vi "inverse se2.vi"(6 "angle unit":u16(ring) items=["radians", "degree"], 8 "error in (no error)":errorcluster, 11 "T":dbl[][](array[numeric])) -> (0 "Error Out":errorcluster, 1 "theta":dbl, 2 "y":dbl, 3 "x":dbl)   [LabVIEW 2017]
doc: "This function builds and outputs a 3x3 homogeneous transformation as a 2-D array(T). Inputs are horizontal translation (X), vertical translation (Y), and rotation (theta) in radians. The default value of theta is 0 rad."
uses:
  <vilib>/Utility/error.llb/Error Cluster From Error Code.vi
  <vilib>/ErrorRing/Error Ring.xnode
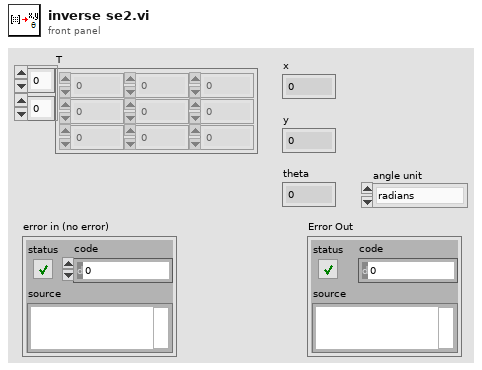
[diagram p1: front panel]
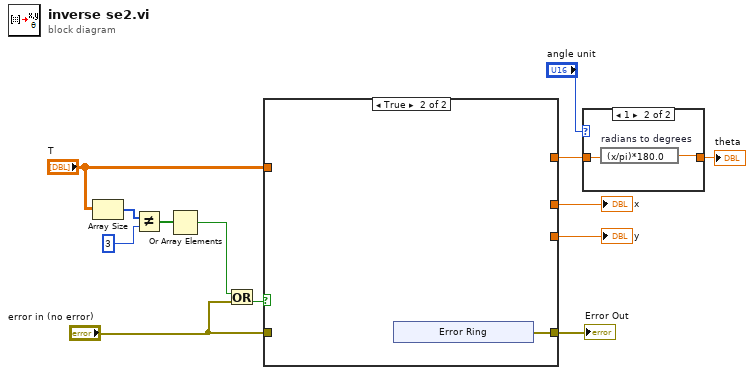
[diagram p0: block diagram]
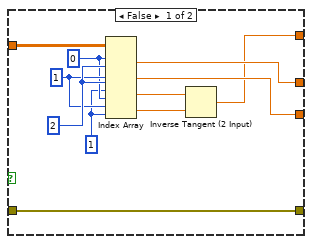
[diagram p3: hidden frame]
diagram:
  n1 = Array Size(array="T") -> (size(s)=w10:i32[])
  n2 = Not Equal?(x=w10, y=3) -> (x != y?=w7:bool[])
  n3 = Or Array Elements(Boolean array=w7) -> (logical OR=w2:bool)
  n4 = Or(x=w2, y="error in (no error)") -> (x .or. y?=w8:bool)
  n5 = case shown="True" w8 {
    tunnel: [w20 w25] -> w13
    tunnel: "T" -> [w24 _]
    tunnel: [w23 _] -> w5
    tunnel: [w21 _] -> w4
    tunnel: "error in (no error)" -> [w20 _]
    tunnel: [w19 _] -> w1
    frame False {
      w14 = 1 ("index (row)")
      w18 = 1 ("index (row)")
      w15 = 0 ("disabled index (row)")
      w22 = 2 ("index (row)")
      n6 = Index Array(array=w24, index (row) #1=w15, index (col) #1=w22, index (row) #2=w18, index (col) #2=w22, index (row) #3=w14, index (col) #3=w15, index (row) #4=w18, index (col) #4=w14) -> (element #1=w23:dbl, element #2=w21:dbl, element #3=w17:dbl, element #4=w16:dbl)
      n7 = Inverse Tangent (2 Input)(1:w16, 2:w17) -> (0:w19:dbl)
    }
    frame True {
      n8 = xnode "Error Ring"() -> ("error out"=w25:errorcluster)
    }
  }
  "x" <- w5
  "y" <- w4
  "Error Out" <- w13
  n9 = case shown="1" "angle unit" {
    tunnel: [w31 w32] -> w11
    tunnel: w1 -> [w31 w33]
    frame 0, Default {
    }
    frame 1 {
      n10 = expression code="(x/pi)*180.0" "radians to degrees"(w33) -> (w32:dbl)
    }
  }
  "theta" <- w11
